vi "createUserEvents.vi"(8 "error in (no error)":errorcluster, 11 "Boot in":refnum<class "Boot.lvclass">) -> (0 "error out":errorcluster, 2 "UserEvents":refnum<class "UserEvents.lvclass">, 3 "Boot out":refnum<class "Boot.lvclass">)   [LabVIEW 2016, in "Boot.lvclass"]
uses:
  Boot.lvclass
  UserEvents/UserEvents.lvclass
  Boot.lvclass/Boot.ctl
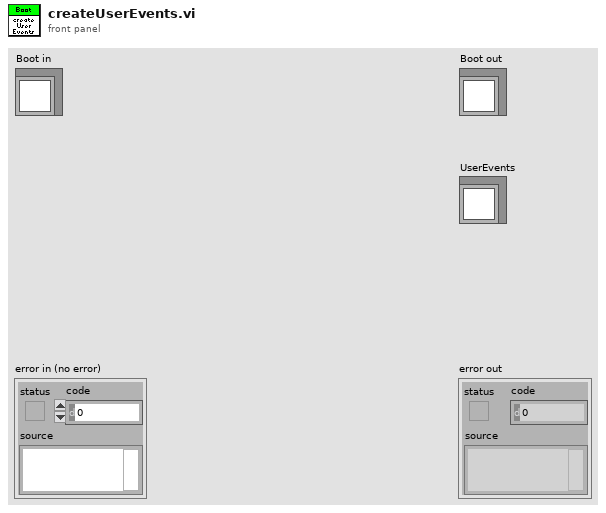
[diagram p1: front panel]
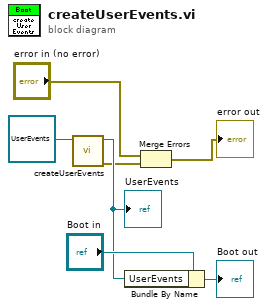
[diagram p0: block diagram]
diagram:
  n1 = call "createUserEvents.vi"("UserEvents in"=refnum<class "UserEvents.lvclass"> refnum ("UserEvents.lvclass")) -> ("error out"=w3:errorcluster, "UserEvents out"=w4:refnum<class "UserEvents.lvclass">)  [unwired: 9 in]
  "UserEvents" <- w4
  n2 = Bundle By Name(cluster="Boot in", "UserEvents"=w4) -> (→"Boot out":refnum<class "Boot.lvclass">)
  n3 = Merge Errors("error in (no error)", w3) -> (→"error out":errorcluster)
